vi "create_channels_AI.vi"(0 "task in":refnum<k21>, 11 "error in":errorcluster) -> (4 "task out":refnum<k21>, 15 "error out":errorcluster)   [LabVIEW 2016]
uses:
  <vilib>/DAQmx/create/scale.llb/DAQmx Create Scale (Linear).vi
  <vilib>/DAQmx/create/channels.llb/DAQmx Create Channel (AI-Voltage-Basic).vi
panel:
  in  "y-intercept":dbl[](array[numeric])=[32.0, 32.0, 32.0, 32.0]
  in  "slope":dbl[](array[numeric])=[4.0, 4.0, 4.0, 4.0]
  in  "maximum":dbl[](array[numeric])=[52.0, 52.0, 52.0, 52.0]
  in  "minimum":dbl[](array[numeric])=[12.0, 12.0, 12.0, 12.0]
  in  "input terminal configuration":i32[](array[ring])=[10083, 10083, 10083, 10083] items=["default"=-1, "RSE"=10083, "NRSE"=10078, "Differential"=10106, "Pseudodifferential"=12529]
  in  "AI lick":tag[](array[tag])=["Dev1/ai4", "Dev1/ai5", "Dev1/ai20", "Dev1/ai21"]
  in  "AI temperature":tag[](array[tag])=["Dev1/ai6", "Dev1/ai7", "Dev1/ai22", "Dev1/ai23"]
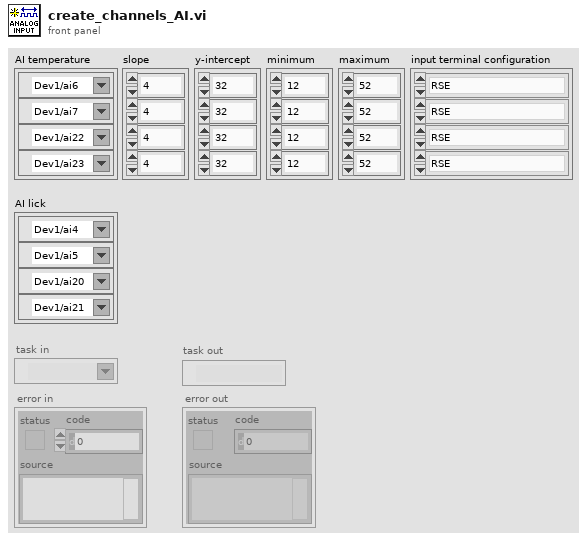
[diagram p1: front panel]
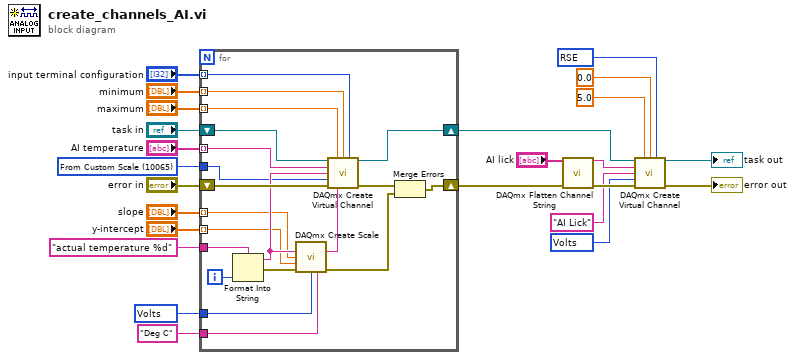
[diagram p0: block diagram]
diagram:
  w1 = 10065 items=["Volts"=10348, "From Custom Scale"=10065] ("units")
  w13 = 10348 items=["Volts"=10348, "Amps"=10342, "Deg F"=10144, "Deg C"=10143, "Deg R"=10145, "Kelvins"=10325, "Strain"=10299, "Ohms"=10384, "Hz"=10373, "Seconds"=10364, "Meters"=10219, "Inches"=10379, "Degrees"=10146, "Radians"=10273, "Ticks"=10304, "g"=10186, "m/s^2"=12470, "m/s"=15959, "in/s"=15960, "Pascals"=10081, "Newtons"=15875, "Pounds"=15876, "kgf"=15877, "psi"=15879, "bar"=15880, "Nm"=15881, "oz-in"=15882, "lb-in"=15883, "lb-ft"=15884, "Volts/Volt"=15896, "mVolts/Volt"=15897, "From TEDS"=12516] ("pre-scaled units")
  w17 = 10348 items=["Volts"=10348, "From Custom Scale"=10065] ("units")
  w18 = 10083 items=["default"=-1, "RSE"=10083, "NRSE"=10078, "Differential"=10106, "Pseudodifferential"=12529] ("input terminal configuration")
  n1 = for {
    tunnel: "AI temperature" -> [w44] mode=indexing
    shift-right: [w43] -> w3
    shift-left: "task in" -> [w42]
    tunnel: w13 -> [w40]
    tunnel: "Deg C" ("scaled units") -> [w39]
    shift-right: [w36] -> w2
    shift-left: "error in" -> [w35]
    tunnel: "maximum" -> [w34] mode=indexing
    tunnel: "minimum" -> [w33] mode=indexing
    tunnel: "input terminal configuration" -> [w32] mode=indexing
    tunnel: "actual temperature %d" ("name") -> [w28]
    tunnel: "y-intercept" -> [w27] mode=indexing
    tunnel: "slope" -> [w26] mode=indexing
    tunnel: w1 -> [w25]
    i -> [w30]
    n2 = Format Into String(format string=w28, w30) -> (resulting string=w29:string, error out=w31:errorcluster)  [unwired: 2 in]
    n3 = call-poly <vilib>:"DAQmx Create Scale.vi"("name"=w29, "slope"=w26, "y-intercept"=w27, "error in"=w31, "pre-scaled units"=w40, "scaled units"=w39) -> ("scale out"=w41:tag, "error out"=w37:errorcluster)  [unwired: 8 in]
    n4 = call-poly <vilib>:"DAQmx Create Virtual Channel.vi"("task in"=w42, "maximum value"=w34, "minimum value"=w33, "input terminal configuration"=w32, "physical channels"=w44, "name to assign"=w29, "units"=w25, "error in"=w35, "custom scale name"=w41) -> ("task out"=w43:refnum<k21>, "error out"=w38:errorcluster)  [unwired: 5 in]
    n5 = Merge Errors(w38, w37) -> (w36:errorcluster)
  }
  n6 = call <vilib>:"DAQmx Flatten Channel String.vi"("names in"="AI lick", "error in"=w2) -> ("names out"=w21:string, "error out"=w24:errorcluster)  [unwired: 12 in]
  n7 = call-poly <vilib>:"DAQmx Create Virtual Channel.vi"("task in"=w3, "maximum value"=5.0, "minimum value"=0.0, "input terminal configuration"=w18, "physical channels"=w21, "name to assign"="AI Lick", "units"=w17, "error in"=w24) -> ("task out"=→"task out":refnum<k21>, "error out"=→"error out":errorcluster)  [unwired: 6 in]
